vi "macro_ReadPathFileWriteTrajectoryCSVFile.vi"() -> ()   [LabVIEW 2019]
uses:
  <vilib>/Rock Robotics/WPI/ThirdParty/JAS_Junk/TrajLib/Trajectory_Library.lvlib
  <vilib>/Rock Robotics/WPI/ThirdParty/JAS_Junk/TrajLib/TypeDef/TRANSLATION2D.ctl
  <vilib>/Rock Robotics/WPI/ThirdParty/JAS_Junk/TrajLib/TypeDef/ROTATION2D.ctl
  TypeDef/PathPlannerPathConstraints.ctl
  TypeDef/PathPlannerTrajectoryState.ctl
  TypeDef/PathPlannerTrajectory.ctl
panel:
  out "Trajectory\nWrite error":errorcluster
  out "Path read\nerror":errorcluster
  out "PathPlannerTrajectory":T1 {"States"."TargetHolonomicRotation"."SIN" format="%13.4f"; "States"."TargetHolonomicRotation"."COS" format="%13.4f"; "States"."TargetHolonomicRotation"."VALUE" format="%13.4f"; "States"."Heading"."SIN" format="%13.4f"; "States"."Heading"."COS" format="%13.4f"; "States"."Heading"."VALUE" format="%13.4f"; "States"."PositionMeters"."Y" format="%14.3f"; "States"."PositionMeters"."X" format="%14.3f"}
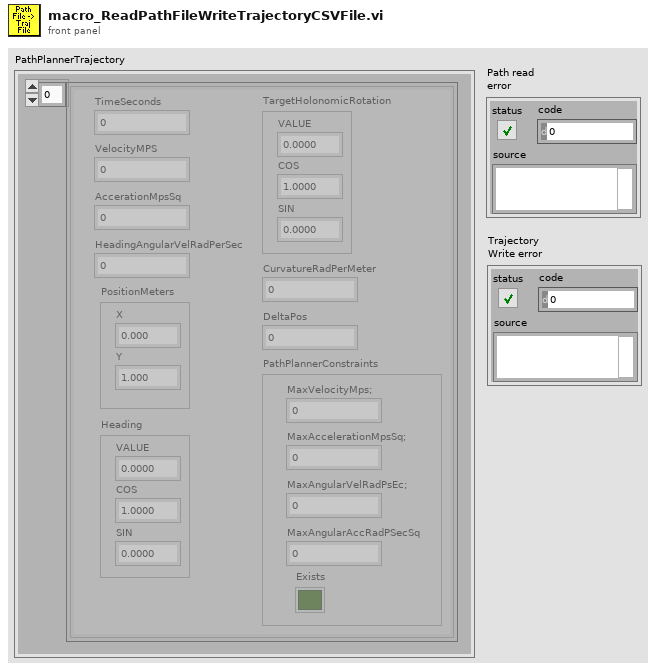
[diagram p1: front panel]
types:
  T1 = typedef "PathPlannerTrajectory.ctl" = cluster{"States":T2[]}
  T2 = typedef "PathPlannerTrajectoryState.ctl" = cluster{"TimeSeconds":dbl, "VelocityMPS":dbl, "AccerationMpsSq":dbl, "HeadingAngularVelRadPerSec":dbl, "PositionMeters":T3, "Heading":T4, "TargetHolonomicRotation":T4, "CurvatureRadPerMeter":dbl, "PathPlannerConstraints":T5, "DeltaPos":dbl}
  T3 = typedef "Trajectory_Library.lvlib/TRANSLATION2D.ctl" = cluster{"X":dbl, "Y":dbl}
  T4 = typedef "Trajectory_Library.lvlib/ROTATION2D.ctl" = cluster{"VALUE":dbl, "COS":dbl, "SIN":dbl}
  T5 = typedef "PathPlannerPathConstraints.ctl" = cluster{"MaxVelocityMps;":dbl, "MaxAccelerationMpsSq;":dbl, "MaxAngularVelRadPsEc;":dbl, "MaxAngularAccRadPSecSq":dbl, "Exists":bool}
  T6 = typedef "Trajectory_Library.lvlib/CHASSIS_SPEEDS.ctl" = cluster{"vX":dbl, "vY":dbl, "vOmega":dbl}
  T7 = typedef "PathPlannerPath.ctl" = cluster{"BezierPoints":T3[], "PreviewStartingRotation":T4, "Reversed":bool, "RotationTargets":T8[], "ConstraintZones":T9[], "EventMarkers":T10[], "GlobalConstraints":T5, "GoalEndState":T13, "AllPoints":T14[]}
  T8 = typedef "PathPlannerRotationTarget.ctl" = cluster{"target":T4, "WaypointRelativePosition":dbl, "Exists":bool}
  T9 = typedef "PathPlannerConstraintsZone.ctl" = cluster{"minWaypointPos":dbl, "maxWaypointPos":dbl, "Constraints":T5, "Present":bool}
  T10 = typedef "PathPlannerEventMarker.ctl" = cluster{"WaypointRelativePos":dbl, "minimumTriggerDistance":dbl, "markerPos":T3, "lastRobotPos":T3, "Command":T11, "markerPos Exists":bool, "LastRobotPoseExists":bool}
  T11 = typedef "PathPlannerCommandUtil.ctl" = cluster{"waitTime":dbl, "name":string, "pathName":string, "commands":cluster{"type":T12, "waitTime":dbl, "name":string, "pathName":string}[], "type":T12}
  T12 = typedef "PathPlanner_CommandUtilType_ENUM.ctl" = enum16{"Unknown", "Wait", "Named", "Path", "Sequential", "Parallel", "Race", "Deadline"}
  T13 = typedef "PathPlannerGoalEndState.ctl" = cluster{"Velocity":dbl, "Rotation":T4}
  T14 = typedef "PathPlannerPathPoint.ctl" = cluster{"Position":T3, "HolonomicRotation":T4, "DistAlongPath":dbl, "CurveRadius":dbl, "MaxV":dbl, "Constraints":T5, "HolonomicRotationExists":bool}
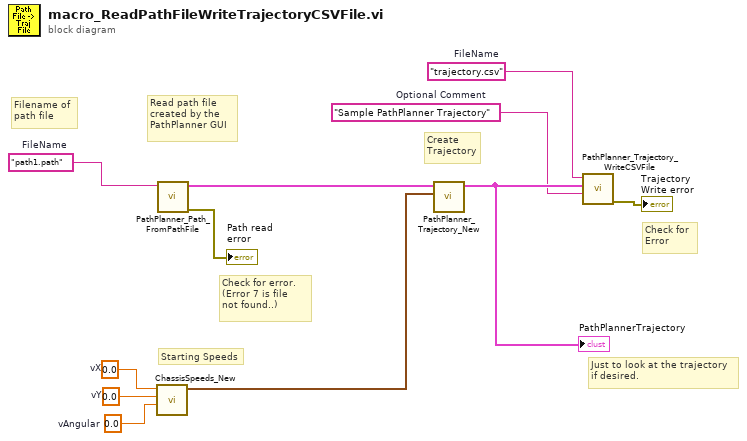
[diagram p0: block diagram]
diagram:
  w2 = "Sample PathPlanner Trajectory"  # Optional Comment
  w4 = "trajectory.csv"  # FileName
  w7 = "path1.path"  # FileName
  w9 = 0.0  # vX
  w10 = 0.0  # vY
  w11 = 0.0  # vAngular
  # "Just to look at the trajectory\nif desired."
  # "Check for\nError"
  # "Check for error.  \n(Error 7 is file\nnot found..)"
  # "Read path file\ncreated by the\nPathPlanner GUI"
  # "Filename of\npath file"
  # "Create\nTrajectory"
  # "Starting Speeds"
  n1 = call <vilib>:"ChassisSpeeds_New.vi"("vAngular"=w11, "vY"=w10, "vX"=w9) -> ("CHASSIS"=w8:T6)  [unwired: 8 in]
  n2 = call "PathPlanner_Path_FromPathFile.vi"("FileName"=w7) -> ("error out"=→"Path read\nerror":errorcluster, "PathPlannerPath"=w6:T7)  [unwired: 8 in, 1 out]
  n3 = call "PathPlanner_Trajectory_New.vi"("StartingSpeeds"=w8, "Path"=w6) -> ("PathPlannerTrajectory"=w3:T1)  [unwired: 9 in]
  "PathPlannerTrajectory" <- w3
  n4 = call "PathPlanner_Trajectory_WriteCSVFile.vi"("Comment"=w2, "TRAJECTORY"=w3, "FileName"=w4) -> ("error out"=→"Trajectory\nWrite error":errorcluster)  [unwired: 8 in]
